vi "XYZToggleJog (SubVI).vi"(0 "Aerotech in":refnum<k24>, 1 "Motion direction":string, 3 "Start location":T1={"X [mm]"=0.001, "Y [mm]"=0.001, "Z [mm]"=0.001}, 5 "Jog step size":T1={"X [mm]"=0.001, "Y [mm]"=0.001, "Z [mm]"=0.001}, 9 "Axis Speeds":T2={"X [mm/s]"=10.0, "Y [mm/s]"=10.0, "Z [mm/s]"=10.0}, 11 "error in (no error)":errorcluster) -> (4 "Aerotech out":refnum<k24>, 6 "Current stage position [mm]":cluster{"X":dbl, "Y":dbl, "Z":dbl}, 8 "completed":bool, 10 "Confirmed location":bool, 15 "error out":errorcluster)   [LabVIEW 2017]
uses:
  <vilib>/regexp/Match Regular Expression.xnode
panel:
  out "done!":bool
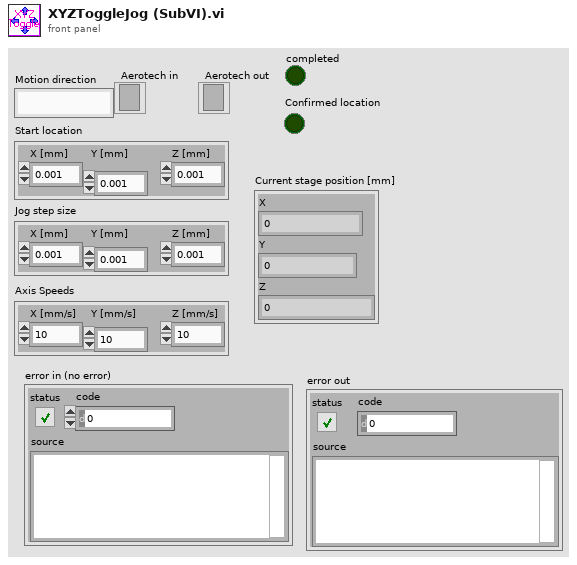
[diagram p1: front panel]
types:
  T1 = cluster{"X [mm]":dbl, "Y [mm]":dbl, "Z [mm]":dbl}
  T2 = cluster{"X [mm/s]":dbl, "Y [mm/s]":dbl, "Z [mm/s]":dbl}
  T3 = cluster{"Final X":dbl, "Final Y":dbl, "Final Z":dbl}
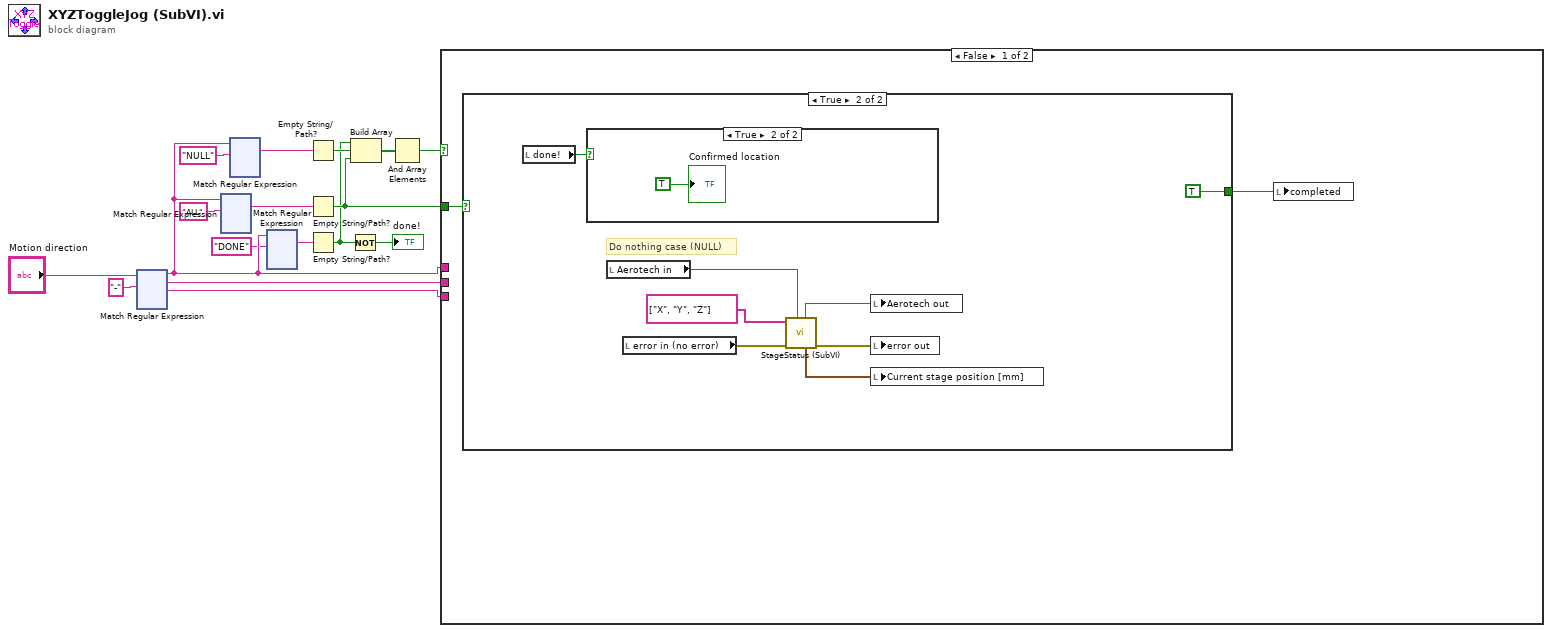
[diagram p0: block diagram]
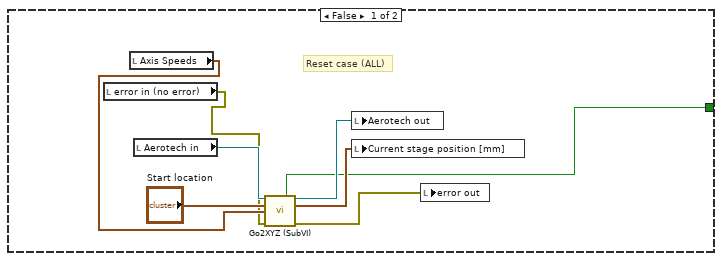
[diagram p2: hidden frame]
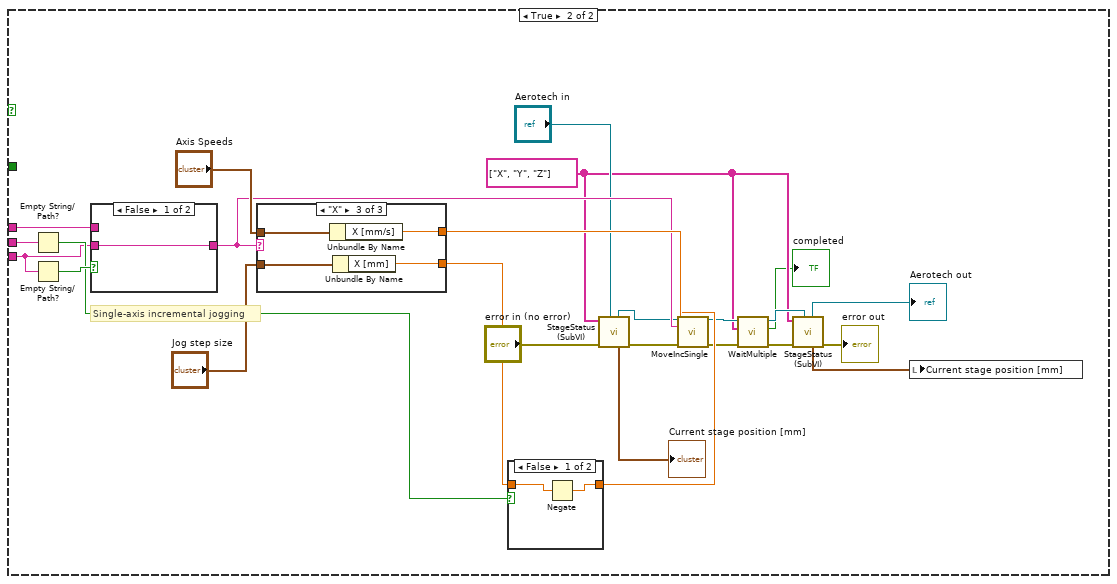
[diagram p4: hidden frame]
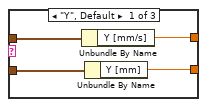
[diagram p7: hidden frame]
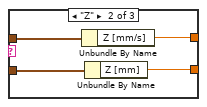
[diagram p8: hidden frame]
diagram:
  n1 = xnode "Match Regular Expression"("input string"="Motion direction", "regular expression"="-") -> ("before match"=w9:string, "whole match"=w15:string, "after match"=w14:string)  [unwired: 4 in, 2 out]
  n2 = xnode "Match Regular Expression"("input string"=w9, "regular expression"="ALL") -> ("whole match"=w12:string)  [unwired: 4 in, 4 out]
  n3 = xnode "Match Regular Expression"("input string"=w9, "regular expression"="NULL") -> ("whole match"=w10:string)  [unwired: 4 in, 4 out]
  n4 = xnode "Match Regular Expression"("input string"=w9, "regular expression"="DONE") -> ("whole match"=w7:string)  [unwired: 4 in, 4 out]
  n5 = Empty String/Path?(string/path=w10) -> (empty?=w6:bool)
  n6 = Empty String/Path?(string/path=w12) -> (empty?=w5:bool)
  n7 = Empty String/Path?(string/path=w7) -> (empty?=w2:bool)
  n8 = Not(x=w2) -> (.not. x?=→"done!":bool)
  n9 = Build Array(w2, w6, w5) -> (w4:bool[])
  n10 = And Array Elements(Boolean array=w4) -> (logical AND=w3:bool)
  n11 = case shown="False" w3 {
    tunnel: w15 -> [_ w52]
    tunnel: w14 -> [_ w51]
    tunnel: w9 -> [_ w50]
    tunnel: w5 -> [w19 _]
    frame False {
      n12 = case shown="True" w19 {
        tunnel: [w20 TRUE ("completed")] -> w18
        frame False {
          # "Reset case (ALL)"
          n13 = local read "error in (no error)"() -> (w21:errorcluster)
          n14 = local read "Axis Speeds"() -> (w27:T2)
          n15 = local read "Aerotech in"() -> (w26:refnum<k24>)
          n16 = call "Go2XYZ (SubVI).vi"(".NET Refnum in"=w26, "Go to Coordinates"="Start location", "Axis Speeds"=w27, "error in (no error)"=w21) -> ("completed"=w20:bool, ".NET Refnum out"=w25:refnum<k24>, "Final Position"=w24:T3, "error out"=w22:errorcluster)  [unwired: 7 in, 1 out]
          n17 = local write "Aerotech out"(w25) -> ()
          n18 = local write "Current stage position [mm]"(w24) -> ()
          n19 = local write "error out"(w22) -> ()
        }
        frame True {
          # "Do nothing case (NULL)"
          n20 = local read "done!"() -> (w28:bool)
          n21 = case shown="True" w28 {
            frame False {
            }
            frame True {
              "Confirmed location" <- TRUE ("Confirmed location")
            }
          }
          n22 = local read "Aerotech in"() -> (w32:refnum<k24>)
          n23 = local read "error in (no error)"() -> (w31:errorcluster)
          n24 = call "StageStatus (SubVI).vi"("Aerotech reference IN"=w32, "error in (no error)"=w31, "Axes Names"=string[] ["X", "Y", "Z"]) -> ("error out"=w30:errorcluster, "Current stage position"=w34:T1, "Aerotech reference OUT"=w33:refnum<k24>)  [unwired: 2 in, 4 out]
          n25 = local write "Aerotech out"(w33) -> ()
          n26 = local write "error out"(w30) -> ()
          n27 = local write "Current stage position [mm]"(w34) -> ()
        }
      }
      n28 = local write "completed"(w18) -> ()
    }
    frame True {
      w38 = string[] ["X", "Y", "Z"] ("Axes Names")
      # "Single-axis incremental jogging"
      n29 = Empty String/Path?(string/path=w52) -> (empty?=w56:bool)
      n30 = Empty String/Path?(string/path=w51) -> (empty?=w57:bool)
      n31 = case shown="False" w57 {
        tunnel: w50 -> [_ w63]
        tunnel: [w62 w63] -> w58
        tunnel: w51 -> [w62 _]
        frame False {
        }
        frame True {
        }
      }
      n32 = case shown="\"X\"" w58 {
        tunnel: [w69 w73 w78] -> w54
        tunnel: [w70 w74 w77] -> w61
        tunnel: "Jog step size" -> [w68 w72 w76]
        tunnel: "Axis Speeds" -> [w67 w71 w75]
        frame "Y", Default {
          n33 = Unbundle By Name(w67) -> ("Y [mm/s]"=w70:dbl)
          n34 = Unbundle By Name(w68) -> ("Y [mm]"=w69:dbl)
        }
        frame "Z" {
          n35 = Unbundle By Name(w71) -> ("Z [mm/s]"=w74:dbl)
          n36 = Unbundle By Name(w72) -> ("Z [mm]"=w73:dbl)
        }
        frame "X" {
          n37 = Unbundle By Name(w75) -> ("X [mm/s]"=w77:dbl)
          n38 = Unbundle By Name(w76) -> ("X [mm]"=w78:dbl)
        }
      }
      n39 = case shown="False" w56 {
        tunnel: w54 -> [w64 w66]
        tunnel: [w65 w66] -> w55
        frame False {
          n40 = Negate(x=w64) -> (-x=w65:dbl)
        }
        frame True {
        }
      }
      n41 = call "StageStatus (SubVI).vi"("Aerotech reference IN"="Aerotech in", "error in (no error)"="error in (no error)", "Axes Names"=w38) -> ("error out"=w48:errorcluster, "Current stage position"=→"Current stage position [mm]":T1, "Aerotech reference OUT"=w46:refnum<k24>)  [unwired: 2 in, 4 out]
      n42 = call "MoveIncSingle.vi"("controller in"=w46, "axis name"=w58, "speed"=w61, "distance"=w55, "error in (no error)"=w48) -> ("controller out"=w40:refnum<k24>, "error out"=w42:errorcluster)  [unwired: 9 in]
      n43 = call "WaitMultiple.vi"("error in (no error)"=w42, "axis names"=w38, "controller in"=w40) -> ("error out"=w41:errorcluster, "completed"=→"completed":bool, "controller out"=w39:refnum<k24>)  [unwired: 6 in]
      n44 = call "StageStatus (SubVI).vi"("Aerotech reference IN"=w39, "error in (no error)"=w41, "Axes Names"=w38) -> ("error out"=→"error out":errorcluster, "Current stage position"=w44:T1, "Aerotech reference OUT"=→"Aerotech out":refnum<k24>)  [unwired: 2 in, 4 out]
      n45 = local write "Current stage position [mm]"(w44) -> ()
    }
  }
